vi "PicoScope4000ExampleRapidBlock.vi"() -> ()   [LabVIEW 2010]
panel:
  out "Capture Complete":bool
  in  "Run":bool
  out "Channel A":i16[][](graph)
  in  "Capture Index":i16 min=0
  in  "Rapid Block Acquisition Settings":T1={"preTriggerSamples"=0, "postTriggerSamples"=1000, "timebase"=2, "Four Channel Device"=FALSE, "Oversample"=1, "Number of Captures"=10}
  in  "Trigger Settings":T2={"Trigger Enabled"=FALSE, "Trigger Source"=enum."Channel A", "Trigger Threshold (16-bit counts)"=0, "Trigger Direction"=2, "Trigger Delay (samples)"=0, "Auto Trigger Time (ms)"=1000} {"Trigger Direction" items=["Rising"=2, "Falling"=3]}
  in  "Channel A Settings":T3={"Enabled"=TRUE, "DC Coupled"=TRUE, "Range"=6} {"Range" items=["10 mV", "20 mV", "50 mV", "100 mV", "200 mV", "500 mV", "1 V", "2 V", "5 V", "10 V", "20 V", "50 V ", "100 V"]}
  in  "stop":bool
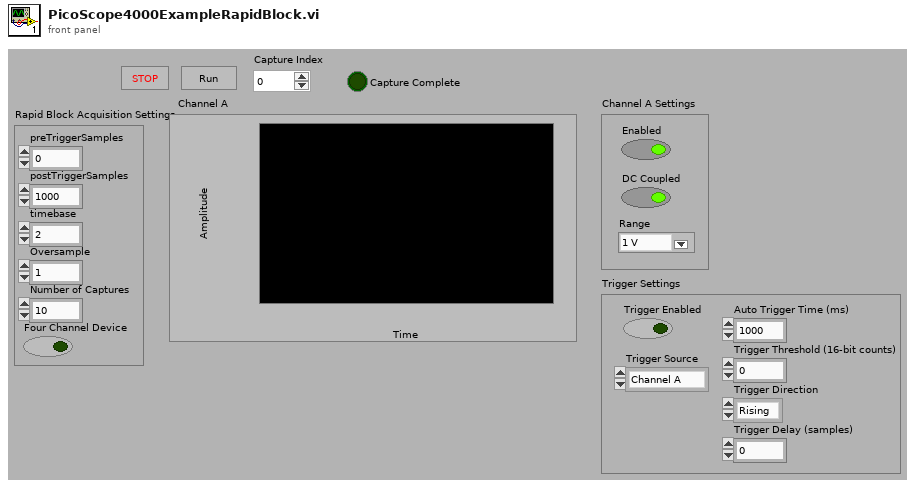
[diagram p1: front panel]
types:
  T1 = cluster{"preTriggerSamples":i32, "postTriggerSamples":i32, "timebase":u32, "Four Channel Device":bool, "Oversample":i16, "Number of Captures":i16}
  T2 = cluster{"Trigger Enabled":bool, "Trigger Source":enum16{"Channel A", "Channel B", "Channel C", "Channel D", "Ext"}, "Trigger Threshold (16-bit counts)":i16, "Trigger Direction":u16, "Trigger Delay (samples)":u32, "Auto Trigger Time (ms)":i16}
  T3 = cluster{"Enabled":bool, "DC Coupled":bool, "Range":u16}
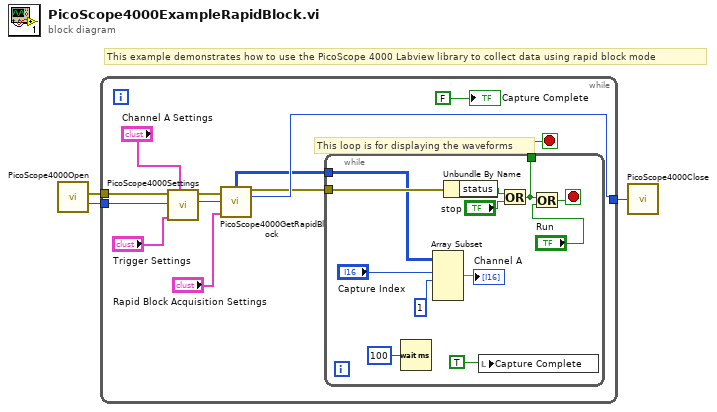
[diagram p0: block diagram]
diagram:
  # "This example demonstrates how to use the PicoScope 4000 Labview library to collect data using rapid block mode"
  n1 = call "PicoScope4000Open.vi"() -> ("error out"=w3:errorcluster, "handle"=w2:i16)  [unwired: 1 in]
  n2 = while {
    tunnel: w2 -> [w15]
    tunnel: w3 -> [w14]
    tunnel: [w8] -> w1
    stop <- w5 stop-if-true
    # "This loop is for displaying the waveforms"
    n3 = call "PicoScope4000Settings.vi"("Channel A Settings"="Channel A Settings", "Trigger Settings"="Trigger Settings", "handle in"=w15, "error in"=w14) -> ("handle out"=w10:i16, "error out"=w9:errorcluster)  [unwired: 6 in]
    n4 = call "PicoScope4000GetRapidBlock.vi"("error in"=w9, "handle in"=w10, "Rapid Block Acquisition Settings"="Rapid Block Acquisition Settings") -> ("Channel A Buffer"=w7:i16[][], "error out"=w6:errorcluster, "handle out"=w8:i16)  [unwired: 7 in, 3 out]
    n5 = while {
      tunnel: w7 -> [w24]
      tunnel: w6 -> [w25]
      tunnel: [w20] -> w5
      stop <- w19 stop-if-true
      n6 = Wait (ms)(milliseconds to wait=u32 100) -> ()  [unwired: 1 out]
      n7 = Array Subset(array=w24, index (row)="Capture Index", length (row)=1 ("length")) -> (→"Channel A":i16[][])  [unwired: 2 in]
      n8 = Unbundle By Name(w25) -> ("status"=w26:bool)
      n9 = local write "Capture Complete"(TRUE ("Capture Complete")) -> ()
      n10 = Or(x=w26, y="stop") -> (x .or. y?=w20:bool)
      n11 = Or(x=w20, y="Run") -> (x .or. y?=w19:bool)
    }
    "Capture Complete" <- FALSE ("Capture Complete")
  }
  n12 = call "PicoScope4000Close.vi"("handle"=w1) -> ()
